vi "Layout - Module Into Subpanel.vi"(7 "SubPanels in":T1, 8 "error in":errorcluster, 10 "VI in":refnum<vi>, 11 "Target SP Name":string) -> (0 "error out":errorcluster, 2 "Removed Module":string, 5 "SubPanels out":T1)   [LabVIEW 2020, in "UI Manager.lvlib"]
doc: "Search <b>SubPanels in</b> Map for the <b>Target SP Name in<b>. If found it check that the <b>VI in</b> reference does not already exist within a subpanel. If all OK it then opens the <b>VI in</b> reference to (Full Delimited Name) and inserts it into target subpanel.. The reference of the inserted VI is placed into the subpanel Map and returned in <b>Subpanels out</b>.\n\nIf either the target subpanel is not found or the VI in is already loaded, an warning message will be logged and the request ignored.\n\n\n\nIf Subpanel VI Ref IN is a valid reference, the front panel of the referenced VI is opened hidden before removing it from the subpanel in order to avoid losing the VI from memory.\n\n\n____\nHAMPEL SOFTWARE ENGINEERING v2.6.0 (2023-12-19 10:54)"
uses:
  UI Manager.lvlib
  SubPanels--map.ctl
  SubPnl Map References--cluster.ctl
  Libraries/hse-libraries/Source/hse-ui/hse-ui.lvlib
  <vilib>/Hampel Software Engineering/HSE Logger/hse-logger.lvlib
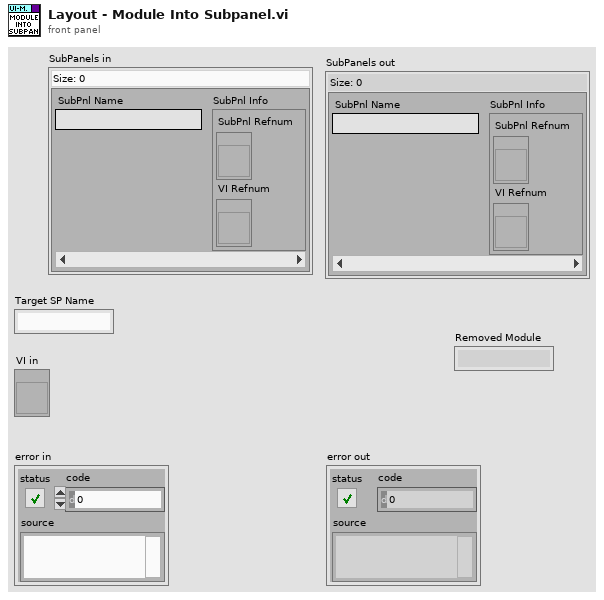
[diagram p1: front panel]
types:
  T1 = typedef "UI Manager.lvlib/SubPanels--map.ctl" = map{string, T2}
  T2 = typedef "UI Manager.lvlib/SubPnl Map References--cluster.ctl" = cluster{"SubPnl Refnum":refnum<vi>, "VI Refnum":refnum<vi>}
  T3 = enum32{"Invalid", "Default", "Floating", "Floating/Auto-Hide", "Modal"}
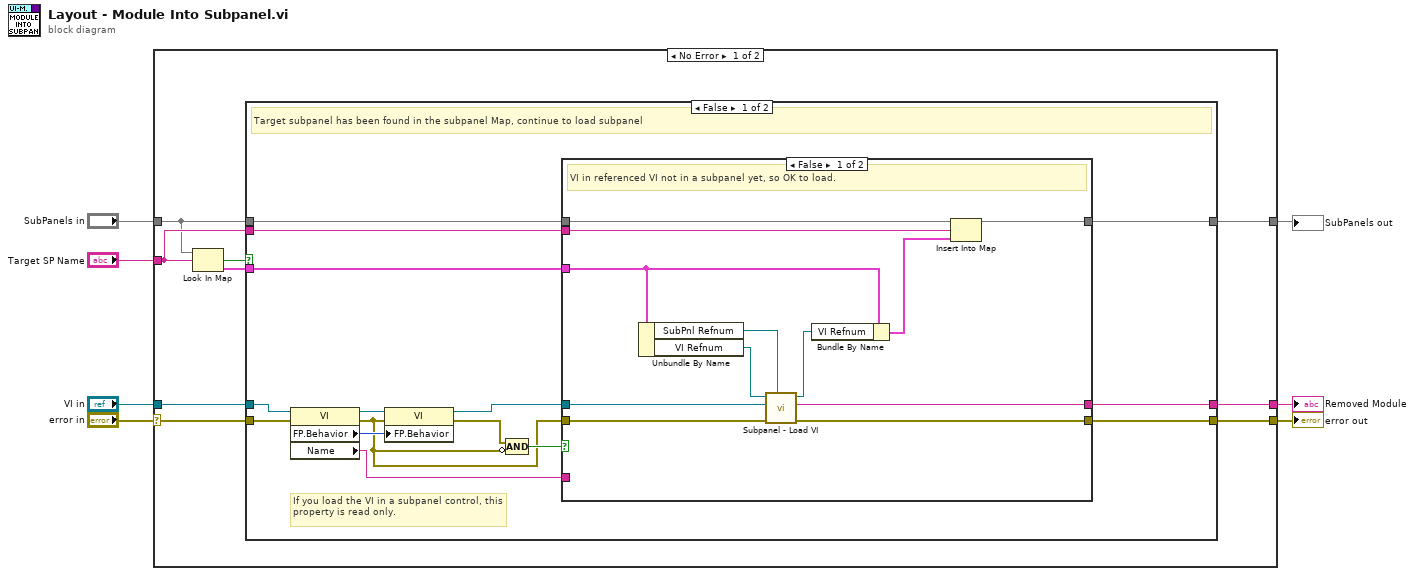
[diagram p0: block diagram]
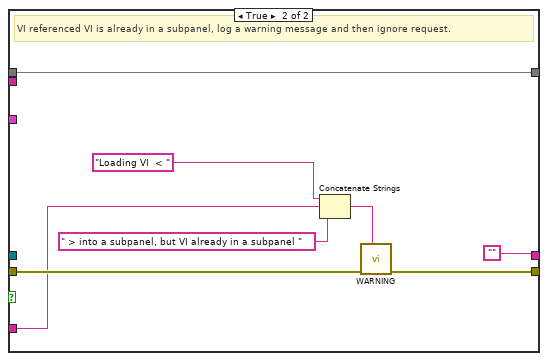
[diagram p2: hidden frame]
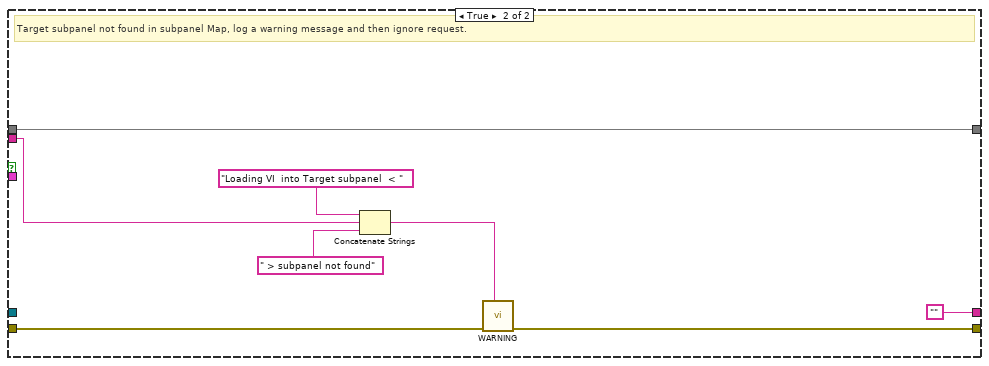
[diagram p3: hidden frame]
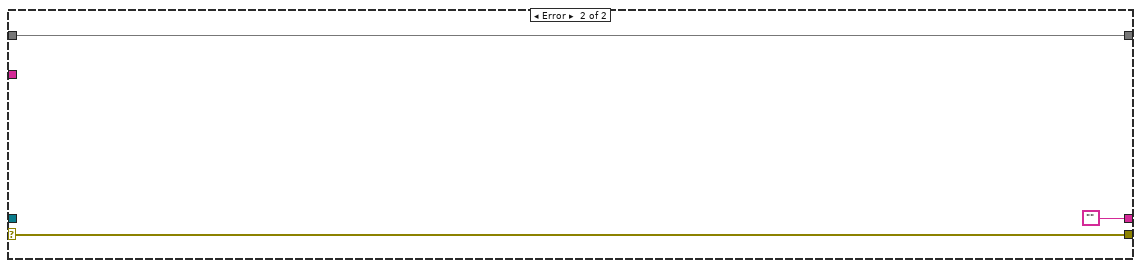
[diagram p4: hidden frame]
diagram:
  n1 = case shown="No Error" "error in" {
    selector: "error in" -> [w8 w61]
    tunnel: "Target SP Name" -> [w15 _]
    tunnel: [w14 w62] -> w6
    tunnel: [w13 w61] -> w5
    tunnel: "VI in" -> [w12 _]
    tunnel: [w11 ""] -> w3
    tunnel: "SubPanels in" -> [w10 w62]
    frame No Error {
      n2 = Look In Map(map=w10, key=w15) -> (key not found?=w9:bool, value=w16:T2)  [unwired: 1 in]
      n3 = case shown="False" w9 {
        tunnel: w16 -> [w31 _]
        tunnel: w15 -> [w30 w53]
        tunnel: [w29 w58] -> w14
        tunnel: [w28 w57] -> w13
        tunnel: w12 -> [w24 _]
        tunnel: [w27 ""] -> w11
        tunnel: w8 -> [w25 w59]
        tunnel: w10 -> [w26 w58]
        frame False {
          # "If you load the VI in a subpanel control, this property is read only."
          # "Target subpanel has been found in the subpanel Map, continue to load subpanel"
          n4 = property class="VI"(reference=w24, error in=w25) -> (reference out=w23:refnum<vi>, error out=w18:errorcluster, "FP.Behavior"=w22:T3, "Name"=w17:string)
          n5 = property class="VI"(reference=w23, error in=w18, "FP.Behavior"=w22) -> (reference out=w21:refnum<vi>, error out=w20:errorcluster)
          n6 = Compound Arithmetic op=AND(w20, invert w18) -> (w19:bool)
          n7 = case shown="False" w19 {
            tunnel: w31 -> [w42 _]
            tunnel: w30 -> [w41 _]
            tunnel: [w39 w48] -> w29
            tunnel: [w38 w50] -> w28
            tunnel: w21 -> [w37 _]
            tunnel: [w36 ""] -> w27
            tunnel: w18 -> [w35 w51]
            tunnel: w26 -> [w33 w48]
            tunnel: w17 -> [_ w46]
            frame False {
              # "VI in referenced VI not in a subpanel yet, so OK to load."
              n8 = Unbundle By Name(w42) -> ("SubPnl Refnum"=w43:refnum<vi>, "VI Refnum"=w32:refnum<vi>)
              n9 = call "Subpanel - Load VI.vi"("SubPanel in"=w43, "error in (no error)"=w35, "VI Reference"=w37, "Subpanel VI Ref IN"=w32) -> ("error out"=w38:errorcluster, "Removed Module"=w36:string, "Subpanel VI Ref OUT"=w34:refnum<vi>)  [unwired: 5 in]
              n10 = Bundle By Name(cluster=w42, "VI Refnum"=w34) -> (w40:T2)
              n11 = Insert Into Map(map in=w33, key=w41, value=w40) -> (map out=w39:T1)  [unwired: 2 out]
            }
            frame True {
              # "VI referenced VI is already in a subpanel, log a warning message and then ignore request."
              n12 = Concatenate Strings("Loading VI  < " ("format string"), w46, " > into a subpanel, but VI already in a subpanel " ("format string")) -> (w44:string)
              n13 = call <vilib>:"WARNING.vi"("Message"=w44, "error in"=w51) -> ("error out"=w50:errorcluster)  [unwired: 9 in]
            }
          }
        }
        frame True {
          # "Target subpanel not found in subpanel Map, log a warning message and then ignore request."
          n14 = Concatenate Strings("Loading VI  into Target subpanel  < " ("format string"), w53, " > subpanel not found" ("format string")) -> (w52:string)
          n15 = call <vilib>:"WARNING.vi"("Message"=w52, "error in"=w59) -> ("error out"=w57:errorcluster)  [unwired: 9 in]
        }
      }
    }
    frame Error {
    }
  }
  "SubPanels out" <- w6
  "error out" <- w5
  "Removed Module" <- w3
